vi "GenNewTraj.vi"(8 "Stoopid Overlap %":dbl min=0.0, 10 "Parameters":T2={"Sample Period (s)"=0.0, "Limits"={"Velocity (fps)"=6.0, "Accel (fps^2)"=15.0, "Jerk (fps^3)"=150.0, "StoopidFast (fps)"=6.0}, "Conditions"={"vInitial (fps)"=0.0, "vFinal (fps)"=0.0}, "Overrides"=[]} {"Overrides"."Angular Multiplier 2" step=5.0; "Overrides"."Angular Multiplier" step=5.0; "Limits"."StoopidFast (fps)" min=0.0; "Limits"."Jerk (fps^3)" min=0.0 step=1.0; "Limits"."Accel (fps^2)" min=0.0; "Limits"."Velocity (fps)" min=0.0}, 11 "Points in":cluster{"x":dbl, "y":dbl, "th":dbl}[](array[cluster])) -> (0 "Time (s)":dbl, 1 "Valid":bool, 2 "Trajectory Data":T3(array[cluster]), 3 "Updated Waypoints":cluster{"x":dbl, "y":dbl, "th":dbl}[](array[cluster]), 4 "Distance (ft)":dbl)   [LabVIEW 2019]
uses:
  Limits.ctl
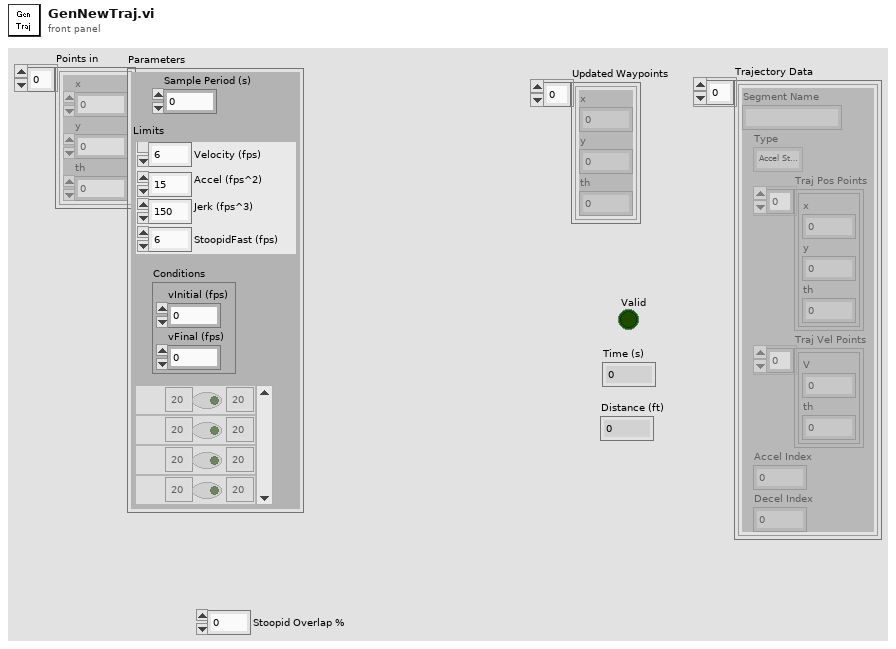
[diagram p1: front panel]
types:
  T1 = typedef "Limits.ctl" = cluster{"Velocity (fps)":dbl, "Accel (fps^2)":dbl, "Jerk (fps^3)":dbl, "StoopidFast (fps)":dbl}
  T2 = cluster{"Sample Period (s)":dbl, "Limits":T1, "Conditions":cluster{"vInitial (fps)":dbl, "vFinal (fps)":dbl}, "Overrides":cluster{"Count":string, "Angular Multiplier":dbl, "1":bool, "Angular Multiplier 2":dbl}[]}
  T3 = cluster{"Segment Name":string, "Type":enum16{"Accel Straight", "Const Straight", "Blend", "Circle"}, "Traj Pos Points":cluster{"x":dbl, "y":dbl, "th":dbl}[], "Traj Vel Points":cluster{"V":dbl, "th":dbl}[], "Accel Index":i32, "Decel Index":i32}[]
  T4 = cluster{"vInitial (fps)":dbl, "vFinal (fps)":dbl}
  T5 = cluster{"Count":string, "Angular Multiplier":dbl, "1":bool, "Angular Multiplier 2":dbl}[]
  T6 = cluster{"Trajectory Data":cluster{"Segment Name":string, "Type":enum16{"Accel Straight", "Const Straight", "Blend", "Circle"}, "Traj Pos Points":cluster{"x":dbl, "y":dbl, "th":dbl}[], "Traj Vel Points":cluster{"V":dbl, "th":dbl}[], "Accel Index":i32, "Decel Index":i32}[], "Time (s)":dbl, "Valid":bool, "Updated Waypoints":cluster{"x":dbl, "y":dbl, "th":dbl}[], "Distance (ft)":dbl}
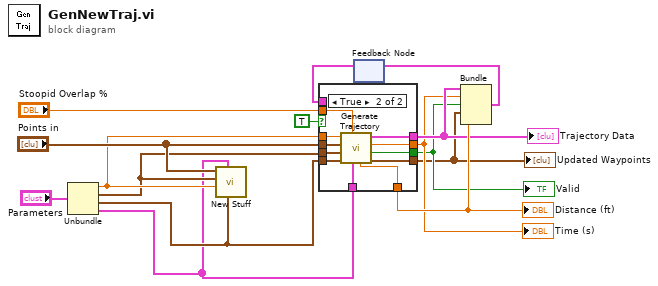
[diagram p0: block diagram]
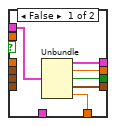
[diagram p2: hidden frame]
diagram:
  n1 = Unbundle("Parameters") -> ("Sample Period (s)"=w6:dbl, "Limits"=w5:T1, "Conditions"=w4:T4, "Overrides"=w1:T5)
  n2 = call "New Stuff.vi"("Conditions"=w4, "Overrides"=w1, "Sample Period (s)"=w6, "Limits"=w5, "Points in"="Points in") -> ()  [unwired: 6 in, 1 out]
  n3 = feedback #1() -> (w13:T6)  [unwired: 1 in]
  n4 = case shown="True" TRUE {
    tunnel: [w18 w32] -> w9
    tunnel: [w19 w31] -> w10
    tunnel: [w16 w30] -> w15
    tunnel: w4 -> [_ w29]
    tunnel: w5 -> [_ w28]
    tunnel: w1 -> [_ w27]
    tunnel: "Points in" -> [_ w26]
    tunnel: [w17 w25] -> w8
    tunnel: [w20 w24] -> w11
    tunnel: w6 -> [_ w23]
    tunnel: w13 -> [w21 _]
    tunnel: "Stoopid Overlap %" -> [_ w22]
    frame False {
      n5 = Unbundle(w21) -> ("Trajectory Data"=w20:T3, "Time (s)"=w19:dbl, "Valid"=w18:bool, "Updated Waypoints"=w17:cluster{"x":dbl, "y":dbl, "th":dbl}[], "Distance (ft)"=w16:dbl)
    }
    frame True {
      n6 = call "Generate Trajectory.vi"("Overrides 2"=w27, "Stoopid Overlap %"=w22, "Conditions"=w29, "Limits"=w28, "WayPoints"=w26, "Sample Period (s)"=w23) -> ("Updated Waypoints"=w25:cluster{"x":dbl, "y":dbl, "th":dbl}[], "Valid"=w32:bool, "Time (s)"=w31:dbl, "Trajectory Data"=w24:T3, "Distance (ft)"=w30:dbl)  [unwired: 1 in]
    }
  }
  "Distance (ft)" <- w15
  "Trajectory Data" <- w11
  "Time (s)" <- w10
  "Valid" <- w9
  "Updated Waypoints" <- w8
  n7 = Bundle("Trajectory Data"=w11, "Time (s)"=w10, "Valid"=w9, "Updated Waypoints"=w8, "Distance (ft)"=w15) -> (w12:T6)  [unwired: 1 in]
  n8 = feedback-in #1(w12) -> ()
